vi "WFT Get Device Name.vi"(8 "Error In":errorcluster, 10 "idxDevice":i32) -> (0 "Error Out":errorcluster, 1 "szDeviceName":string, 2 "ret":i32)   [LabVIEW 2020, in "lv_waveforms_toolkit.lvlib"]
uses:
  lv_waveforms_toolkit.lvlib
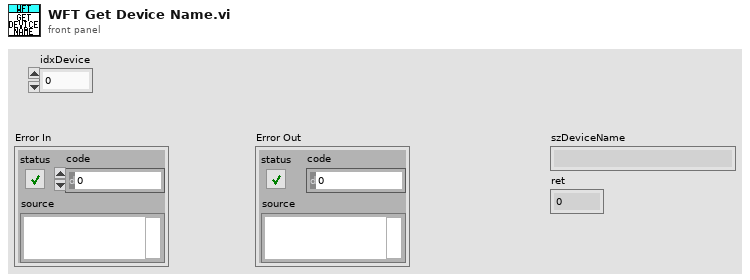
[diagram p1: front panel]
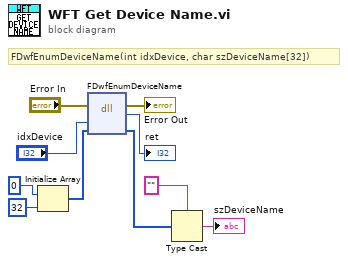
[diagram p0: block diagram]
diagram:
  # "FDwfEnumDeviceName(int idxDevice, char szDeviceName[32])"
  n1 = Initialize Array(u8 0, 32 ("dimension size")) -> (w8:u8[])
  n2 = dll-call lib="dwf" fn="FDwfEnumDeviceName"(error in="Error In", "idxDevice"="idxDevice", "szDeviceName"=w8) -> (error out=→"Error Out":errorcluster, "return type"=→"ret":i32, "szDeviceName"=w7:u8[])  [unwired: 3 in, 1 out]
  n3 = Type Cast(type="", x=w7) -> (*(type *) &x=→"szDeviceName":string)
